vi "GetEnvironmentalVariable-subvi.vi"(2 "Variable name":string) -> (0 "Value":string)   [LabVIEW 2014]
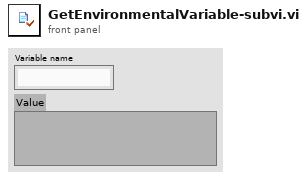
[diagram p1: front panel]
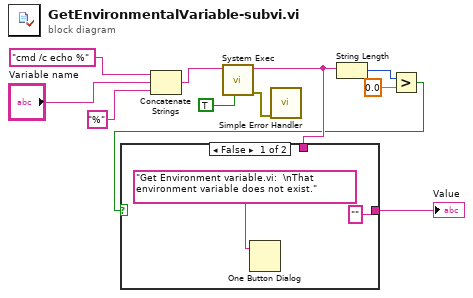
[diagram p0: block diagram]
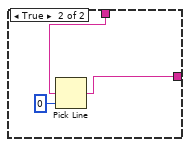
[diagram p2: hidden frame]
diagram:
  n1 = Concatenate Strings("cmd /c echo %", "Variable name", "%") -> (w11:string)
  n2 = call <vilib>:"System Exec.vi"("run minimized? (F)"=TRUE, "command line"=w11) -> ("error out"=w7:errorcluster, "standard output"=w5:string)  [unwired: 4 in, 4 out]
  n3 = call <vilib>:"Simple Error Handler.vi"("error in (no error)"=w7) -> ()  [unwired: 1 in, 8 out]
  n4 = String Length(string=w5) -> (length=w3:i32)
  n5 = Greater?(x=w3, y=0.0) -> (0:w2:bool)
  n6 = case shown="False" w2 {
    tunnel: w5 -> [_ w16]
    tunnel: ["" ("output string") w14] -> w1
    frame False {
      n7 = One Button Dialog(message="Get Environment variable.vi:  \nThat environment variable does not exist.") -> ()  [unwired: 2 out]
    }
    frame True {
      n8 = Pick Line(multi-line string=w16, line index=0) -> (output string=w14:string)  [unwired: 1 out]
    }
  }
  "Value" <- w1
